vi "Create Configuration File.vi"(0 "Config File In":path, 11 "error in (no error)":errorcluster) -> (4 "Config File Out":path, 15 "error out":errorcluster)   [LabVIEW 2021, in "Packager Helpers.lvlib"]
uses:
  Packager Helpers.lvlib
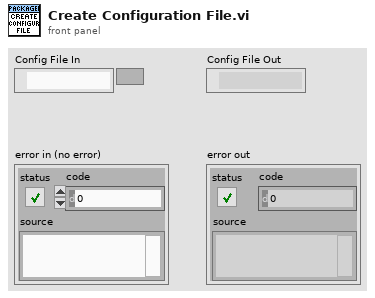
[diagram p1: front panel]
types:
  T1 = enum16{"open", "replace", "create", "open or create", "replace or create", "replace or create with confirmation"}
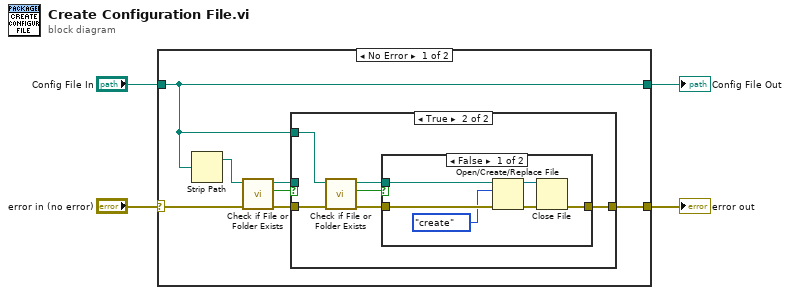
[diagram p0: block diagram]
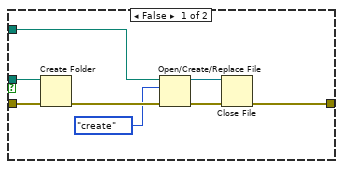
[diagram p2: hidden frame]
diagram:
  n1 = case shown="No Error" "error in (no error)" {
    selector: "error in (no error)" -> [w11 w33]
    tunnel: "Config File In" -> [w5 w34]
    tunnel: [w8 w33] -> w2
    tunnel: [w5 w34] -> w1
    frame No Error {
      n2 = Strip Path(path=w5) -> (stripped path=w10:path)  [unwired: 1 out]
      n3 = call <vilib>:"Check if File or Folder Exists.vi"("error in (no error)"=w11, "path"=w10) -> ("error out"=w9:errorcluster, "file or folder exists?"=w7:bool, "dup path"=w6:path)  [unwired: 7 in]
      n4 = case shown="True" w7 {
        tunnel: w9 -> [w19 w25]
        tunnel: [w14 w23] -> w8
        tunnel: w6 -> [w13 _]
        tunnel: w5 -> [w12 w20]
        frame False {
          n5 = Create Folder(path (use dialog)=w13, error in=w19) -> (error out=w18:errorcluster)  [unwired: 1 in, 2 out]
          n6 = Open/Create/Replace File(file path (use dialog)=w12, error in=w18, operation (0:open)=T1."create") -> (refnum out=w16:refnum<file>, error out=w15:errorcluster)  [unwired: 3 in, 1 out]
          n7 = Close File(refnum=w16, error in=w15) -> (error out=w14:errorcluster)  [unwired: 1 out]
        }
        frame True {
          n8 = call <vilib>:"Check if File or Folder Exists.vi"("error in (no error)"=w25, "path"=w20) -> ("error out"=w24:errorcluster, "file or folder exists?"=w21:bool, "dup path"=w22:path)  [unwired: 7 in]
          n9 = case shown="False" w21 {
            tunnel: w24 -> [w29 w32]
            tunnel: [w28 w32] -> w23
            tunnel: w22 -> [w26 _]
            frame False {
              n10 = Open/Create/Replace File(file path (use dialog)=w26, error in=w29, operation (0:open)=T1."create") -> (refnum out=w31:refnum<file>, error out=w30:errorcluster)  [unwired: 3 in, 1 out]
              n11 = Close File(refnum=w31, error in=w30) -> (error out=w28:errorcluster)  [unwired: 1 out]
            }
            frame True {
            }
          }
        }
      }
    }
    frame Error {
    }
  }
  "error out" <- w2
  "Config File Out" <- w1
